vi "LibXML_SelectNodesInDocument.vi"(8 "error in":errorcluster, 9 "queryString":string, 10 "rootnode (root of doc)":u32, 11 "doc":u32) -> (0 "error out":errorcluster, 1 "NodePtr":u32, 2 "length":i32, 3 "xmlXPathObj":u32, 4 "Not found":bool, 5 "doc copy out":u32)   [LabVIEW 2019, in "Tools.lvlib" / "LibXML.lvlib"]
doc: "This VI searches the XMLDocument with the querystring according to the XPATH protocol and returns the number (length) of the nodes found as well as the first Node found. If not found \"not found\"will be set true"
uses:
  LibXML.lvlib
  Error Cluster From Error Code_subroutine.vi
  <vilib>/Utility/error.llb/Trim Whitespace.vi
panel:
  # "This software is FREE licensed under the GNU Lesser General Public License"
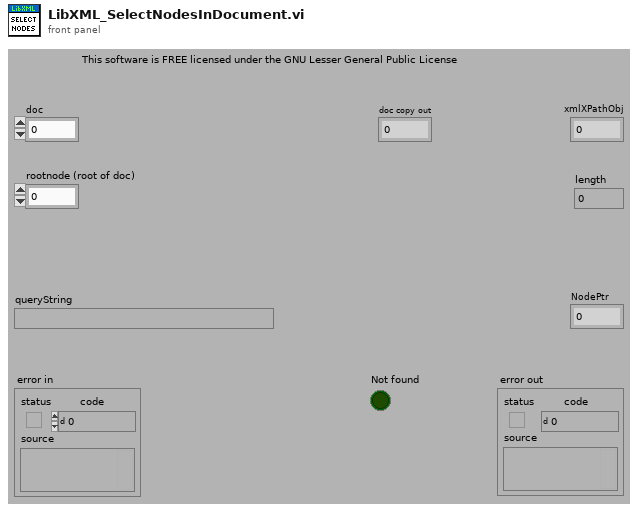
[diagram p1: front panel]
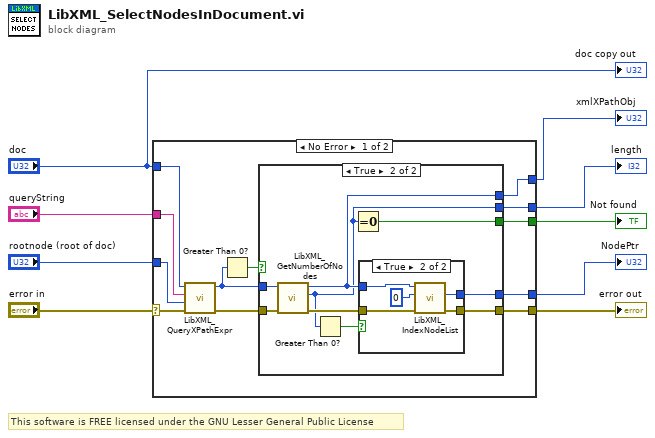
[diagram p0: block diagram]
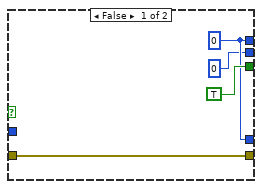
[diagram p2: hidden frame]
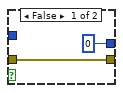
[diagram p3: hidden frame]
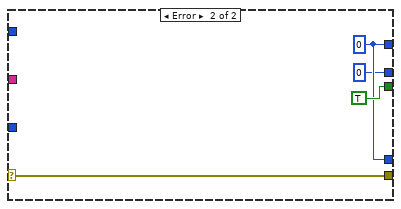
[diagram p4: hidden frame]
diagram:
  # "This software is FREE licensed under the GNU Lesser General Public License"
  n1 = case shown="No Error" "error in" {
    selector: "error in" -> [w21 w45]
    tunnel: [w16 w45] -> w9
    tunnel: "doc" -> [w15 _]
    tunnel: [w19 TRUE ("Not found")] -> w7
    tunnel: [w14 w43] -> w6
    tunnel: [w13 w43] -> w5
    tunnel: [w12 0 ("#ofNodes")] -> w4
    tunnel: "queryString" -> [w11 _]
    tunnel: "rootnode (root of doc)" -> [w10 _]
    frame No Error {
      n2 = call "LibXML_QueryXPathExpr.vi"("error in"=w21, "rootnode (root of doc)"=w10, "XPathExpr"=w11, "doc"=w15) -> ("error out"=w18:errorcluster, "xmlXPathObj"=w17:u32)  [unwired: 6 in]
      n3 = Greater Than 0?(x=w17) -> (x > 0?=w20:bool)
      n4 = case shown="True" w20 {
        tunnel: [TRUE ("Not found") w34] -> w19
        tunnel: w18 -> [w24 w33]
        tunnel: w17 -> [_ w32]
        tunnel: [w24 w29] -> w16
        tunnel: [w23 w28] -> w14
        tunnel: [w23 w27] -> w13
        tunnel: [0 ("#ofNodes") w26] -> w12
        frame False {
          w23 = u32 0 ("XPathObj out")
        }
        frame True {
          n5 = call "LibXML_GetNumberOfNodes.vi"("error in (no error)"=w33, "XPathObj"=w32) -> ("error out"=w30:errorcluster, "#ofNodes"=w26:i32, "XPathObj out"=w27:u32)  [unwired: 7 in]
          n6 = Greater Than 0?(x=w26) -> (x > 0?=w31:bool)
          n7 = Equal To 0?(x=w26) -> (x = 0?=w34:bool)
          n8 = case shown="True" w31 {
            tunnel: w30 -> [w36 w40]
            tunnel: [w36 w39] -> w29
            tunnel: w27 -> [_ w38]
            tunnel: [u32 0 ("NodePtr") w37] -> w28
            frame False {
            }
            frame True {
              n9 = call "LibXML_IndexNodeList.vi"("error in"=w40, "index"=0, "XPathObj"=w38) -> ("error out"=w39:errorcluster, "NodePtr"=w37:u32)  [unwired: 6 in, 1 out]
            }
          }
        }
      }
    }
    frame Error {
      w43 = u32 0 ("XPathObj out")
    }
  }
  "error out" <- w9
  "Not found" <- w7
  "xmlXPathObj" <- w5
  "NodePtr" <- w6
  "length" <- w4
  "doc copy out" <- "doc"
